vi "Configure OCP.vi"(7 "OCP Delay Time Start Type (0: Command Changed)":u16(ring) items=["Command Changed", "Any Transition Method"], 8 "error in (no error)":errorcluster, 9 "OCP Delay Time (0.02)":dbl=0.02, 10 "Enable OCP (F: Disabled)":bool, 11 "VISA resource name":refnum<visa-resource-name>) -> (0 "error out":errorcluster, 3 "VISA resource name out":refnum<visa-resource-name>)   [LabVIEW 2021, in "Agilent N6900 N7900 Series.lvlib"]
doc: "Configures the Over Current Protection settings to protect from a current overload."
uses:
  <instrlib>/Agilent N6900 N7900 Series/Agilent N6900 N7900 Series.lvlib
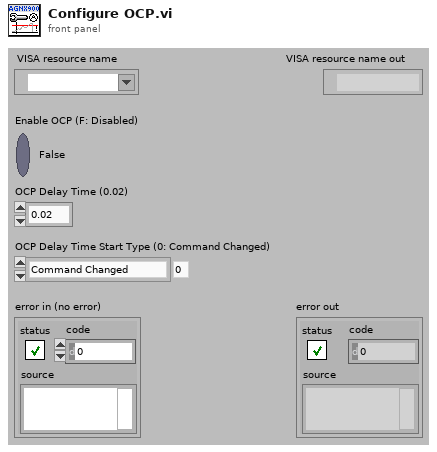
[diagram p1: front panel]
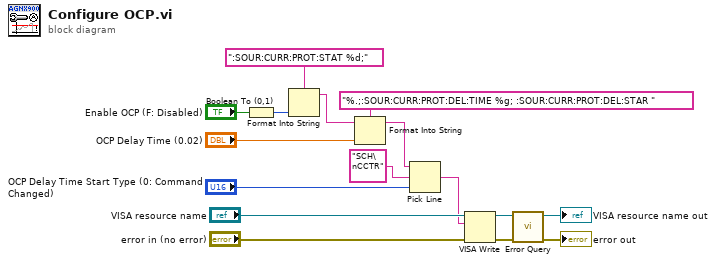
[diagram p0: block diagram]
diagram:
  n1 = Boolean To (0,1)(Boolean="Enable OCP (F: Disabled)") -> (0, 1=w2:i16)
  n2 = Format Into String(format string=":SOUR:CURR:PROT:STAT %d;" ("string (\"\")"), w2) -> (resulting string=w1:string)  [unwired: 2 in, 1 out]
  n3 = Format Into String(format string="%.;:SOUR:CURR:PROT:DEL:TIME %g; :SOUR:CURR:PROT:DEL:STAR ", initial string=w1, "OCP Delay Time (0.02)") -> (resulting string=w7:string)  [unwired: 1 in, 1 out]
  n4 = Pick Line(string ("")=w7, multi-line string="SCH\nCCTR", line index="OCP Delay Time Start Type (0: Command Changed)") -> (output string=w10:string)
  n5 = VISA Write(VISA resource name="VISA resource name", write buffer=w10, error in (no error)="error in (no error)") -> (VISA resource name out=w13:refnum<visa-resource-name>, error out=w14:errorcluster)  [unwired: 1 out]
  n6 = call <instrlib>:"Error Query.vi"("error in (no error)"=w14, "VISA resource name"=w13) -> ("error out"=→"error out":errorcluster, "VISA resource name out"=→"VISA resource name out":refnum<visa-resource-name>)  [unwired: 6 in, 2 out]
